vi "Configure.vi"(8 "error in (no error)":errorcluster, 11 "DAQ_QPT_Throlab in":refnum<class "DAQ_QPT_Throlab.lvclass">) -> (0 "error out":errorcluster, 3 "DAQ_QPT_Throlab out":refnum<class "DAQ_QPT_Throlab.lvclass">)   [LabVIEW 2020, in "DAQ_QPT_Throlab.lvlib" / "DAQ_QPT_Throlab.lvclass"]
uses:
  DAQ_QPT_Throlab.lvclass
  DAQ_QPT_Throlab.lvclass/DAQ_QPT_Throlab.ctl
  Hardware Abstraction Layer/Component/DAQ/DAQ/DAQ.lvclass
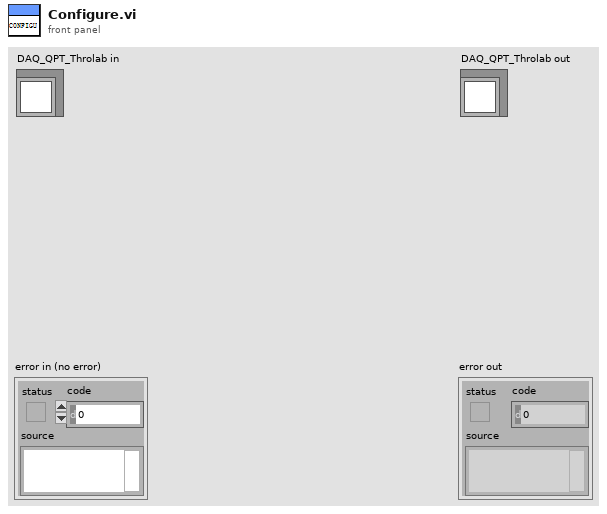
[diagram p1: front panel]
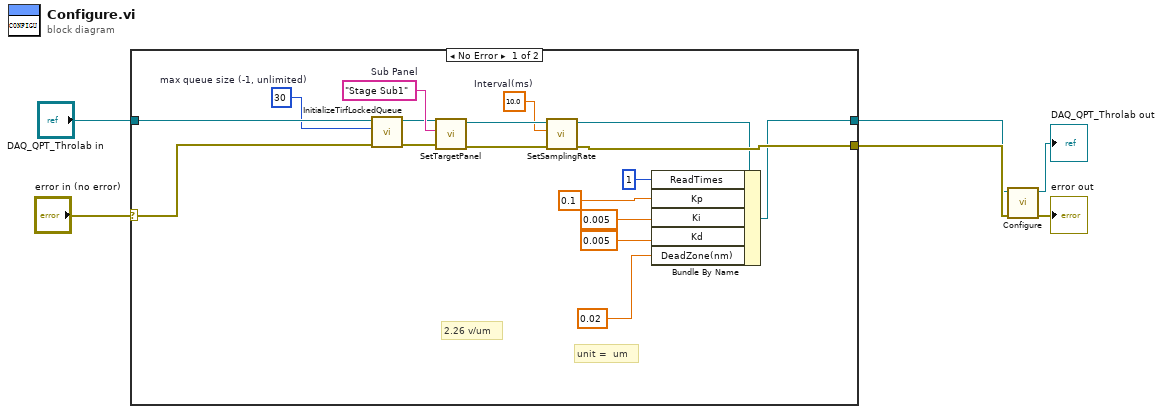
[diagram p0: block diagram]
diagram:
  n1 = case shown="No Error" "error in (no error)" {
    selector: "error in (no error)" -> [w22 w25]
    tunnel: [w19 w25] -> w2
    tunnel: [w12 w24] -> w1
    tunnel: "DAQ_QPT_Throlab in" -> [w23 w24]
    frame No Error {
      w14 = 30  # max queue size (-1, unlimited)
      w17 = 10.0  # Interval(ms)
      w21 = "Stage Sub1"  # Sub Panel
      # "unit =  um"
      # "2.26 v/um"
      n2 = call-dynamic "InitializeTirfLockedQueue.vi"("error in (no error)"=w22, "max queue size (-1, unlimited)"=w14, "DAQ_QPT_Throlab in"=w23) -> ("error out"=w16:errorcluster, "DAQ_QPT_Throlab out"=w15:refnum<class "DAQ_QPT_Throlab.lvclass">)  [unwired: 7 in]
      n3 = call-dynamic "SetTargetPanel.vi"("error in (no error)"=w16, "TargetPanel"=w21, "GRMActor in"=w15) -> ("error out"=w20:errorcluster, "GRMActor out"=w18:refnum<class "DAQ_QPT_Throlab.lvclass">)  [unwired: 7 in]
      n4 = call-dynamic "SetSamplingRate.vi"("error in (no error)"=w20, "SamplingRate(Hz)"=w17, "Device in"=w18) -> ("error out"=w19:errorcluster, "Device out"=w13:refnum<class "DAQ_QPT_Throlab.lvclass">)  [unwired: 7 in]
      n5 = Bundle By Name(cluster=w13, "ReadTimes"=1, "Kp"=0.1 ("PIDParams.Kp"), "Ki"=0.005 ("PIDParams.Ki"), "Kd"=0.005 ("PIDParams.Kd"), "DeadZone(nm)"=0.02 ("PIDParams.DeadZone(nm)")) -> (w12:refnum<class "DAQ_QPT_Throlab.lvclass">)
    }
    frame Error {
    }
  }
  n6 = call-parent "Configure.vi"("error in (no error)"=w2, "Device in"=w1) -> ("error out"=→"error out":errorcluster, "Device out"=→"DAQ_QPT_Throlab out":refnum<class "DAQ_QPT_Throlab.lvclass">)  [unwired: 8 in]
